vi "FMSweep-Create Linear.vi"(0 "Sweep Rate (Hz/s)":dbl=42900000.0, 1 "cal file":path, 5 "Fmin (Hz)":dbl=100.0, 7 "Fmax (Hz)":dbl=60000.0, 9 "Ramp (ms)":dbl=0.1, 11 "error in (no error)":errorcluster, 12 "Fs (Hz)":dbl) -> (8 "Array":dbl[](array[numeric]), 10 "Reference":dbl, 15 "error out":errorcluster)   [LabVIEW 2020]
uses:
  Utility VIs/Math VIs/LinSpace (x0-dx-npts).vi
  <vilib>/Analysis/5stat.llb/RMS (DBL).vi
  Utility VIs/Math VIs/Linear to dB (scalar).vi
  <vilib>/Analysis/NI_AALPro.lvlib
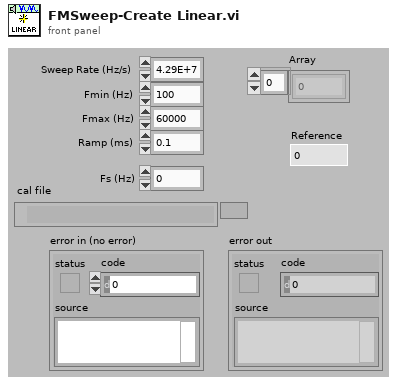
[diagram p1: front panel]
types:
  T1 = cluster{"Active":bool, "Delay (ms)":dbl, "Width (ms)":dbl, "Ramp (ms)":dbl}
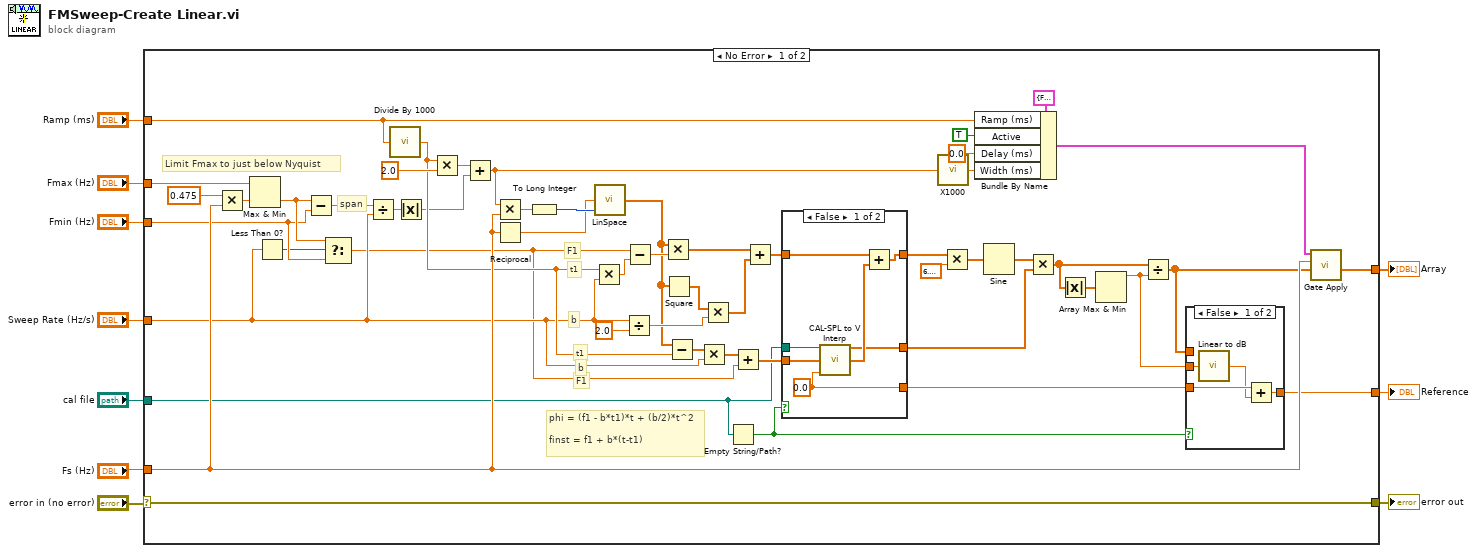
[diagram p0: block diagram]
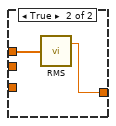
[diagram p2: hidden frame]
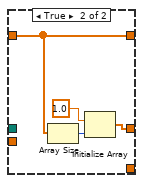
[diagram p3: hidden frame]
diagram:
  n1 = case shown="No Error" "error in (no error)" {
    selector: "error in (no error)" -> [w62 w80]
    tunnel: [w62 w80] -> w9
    tunnel: "Fmax (Hz)" -> [w61 _]
    tunnel: "Fs (Hz)" -> [w42 _]
    tunnel: "Fmin (Hz)" -> [w40 _]
    tunnel: "Sweep Rate (Hz/s)" -> [w27 _]
    tunnel: [w47 _] -> w3
    tunnel: "Ramp (ms)" -> [w38 _]
    tunnel: "cal file" -> [w21 _]
    tunnel: [w14 _] -> w1
    frame No Error {
      # "F1"
      # "b"
      # "t1"
      # "t1"
      # "F1"
      # "b"
      # "Limit Fmax to just below Nyquist"
      # "span"
      # "phi = (f1 - b*t1)*t + (b/2)*t^2\n\nfinst = f1 + b*(t-t1)"
      n2 = Multiply(x=0.475 ("y"), y=w42) -> (x*y=w60:dbl)
      n3 = Max & Min(x=w61, y=w60) -> (min(x,y)=w41:dbl)  [unwired: 1 out]
      n4 = Less Than 0?(x=w27) -> (x < 0?=w39:bool)
      n5 = Subtract(x=w41, y=w40) -> (x-y=w58:dbl)
      n6 = Select(t=w41, s=w39, f=w40) -> (s? t:f=w25:dbl)
      n7 = Divide(x=w58, y=w27) -> (x/y=w34:dbl)
      n8 = call "Divide By 1000.vi"("X"=w38) -> ("X/1000"=w29:dbl)
      n9 = Absolute Value(x=w34) -> (abs(x)=w11:dbl)
      n10 = Multiply(x=w29, y=2.0) -> (x*y=w35:dbl)
      n11 = Add(x=w35, y=w11) -> (x+y=w12:dbl)
      n12 = Multiply(x=w12, y=w42) -> (x*y=w36:dbl)
      n13 = Reciprocal(x=w42) -> (1/x=w56:dbl)
      n14 = To Long Integer(number=w36) -> (32bit integer=w57:i32)
      n15 = Multiply(x=w29, y=w27) -> (x*y=w32:dbl)
      n16 = call-poly "LinSpace.vi"("npts"=w57, "dx"=w56) -> ("Array"=w30:dbl[])  [unwired: 2 in, 1 out]
      n17 = Divide(x=w27, y=2.0) -> (x/y=w54:dbl)
      n18 = Subtract(x=w25, y=w32) -> (x-y=w31:dbl)
      n19 = Multiply(x=w30, y=w31) -> (x*y=w53:dbl[])
      n20 = Square(x=w30) -> (x^2=w55:dbl[])
      n21 = Subtract(x=w30, y=w29) -> (x-y=w28:dbl[])
      n22 = Multiply(x=w28, y=w27) -> (x*y=w26:dbl[])
      n23 = Multiply(x=w55, y=w54) -> (x*y=w52:dbl[])
      n24 = Empty String/Path?(string/path=w21) -> (empty?=w17:bool)
      n25 = Add(x=w26, y=w25) -> (x+y=w24:dbl[])
      n26 = Add(x=w53, y=w52) -> (x+y=w23:dbl[])
      n27 = case shown="False" w17 {
        tunnel: w24 -> [w75 _]
        tunnel: w23 -> [w74 w77]
        tunnel: [w70 w77] -> w22
        tunnel: w21 -> [w72 _]
        tunnel: [w71 w79] -> w20
        tunnel: [w69 _] -> w16
        frame False {
          w69 = 0.0
          n28 = call "CAL-SPL to V Interp.vi"("user path"=w72, "Fi (Hz)"=w75, "dB SPL"=w69) -> ("Amplitude (V)"=w71:dbl[], "Phase (cycles)"=w73:dbl[])  [unwired: 11 in]
          n29 = Add(x=w74, y=w73) -> (x+y=w70:dbl[])
        }
        frame True {
          n30 = Array Size(array=w77) -> (size(s)=w78:i32)
          n31 = Initialize Array(1.0 ("element"), w78) -> (w79:dbl[])
        }
      }
      n32 = call "X1000.vi"("X"=w12) -> ("X/1000"=w43:dbl)
      n33 = Multiply(x=w22, y=6.283185307179586) -> (x*y=w50:dbl[])
      n34 = Bundle By Name(cluster=T1 {"Active"=FALSE, "Delay (ms)"=0.0, "Width (ms)"=0.0, "Ramp (ms)"=0.0} ("Gate Control"), "Ramp (ms)"=w38, "Active"=TRUE, "Delay (ms)"=0.0, "Width (ms)"=w43) -> (w46:T1)
      n35 = Sine(x=w50) -> (sin(x)=w49:dbl[])
      n36 = Multiply(x=w49, y=w20) -> (x*y=w19:dbl[])
      n37 = Absolute Value(x=w19) -> (abs(x)=w18:dbl[])
      n38 = Array Max & Min(array=w18) -> (max value=w15:dbl)  [unwired: 3 out]
      n39 = Divide(x=w19, y=w15) -> (x/y=w13:dbl[])
      n40 = case shown="False" w17 {
        tunnel: w16 -> [w65 _]
        tunnel: w15 -> [w66 _]
        tunnel: [w63 w67] -> w14
        tunnel: w13 -> [_ w68]
        frame False {
          n41 = call-poly "Linear to dB.vi"("Linear"=w66) -> ("dB"=w64:dbl)
          n42 = Add(x=w65, y=w64) -> (x+y=w63:dbl)
        }
        frame True {
          n43 = call-poly <vilib>:"RMS.vi"("X"=w68) -> ("rms value"=w67:dbl)  [unwired: 1 out]
        }
      }
      n44 = call "Gate Apply.vi"("Waveform in"=w13, "Sampling Rate (Hz)"=w42, "Gate Control"=w46) -> ("Gated waveform"=w47:dbl[])  [unwired: 7 in, 1 out]
    }
    frame Error {
    }
  }
  "error out" <- w9
  "Array" <- w3
  "Reference" <- w1
